vi "Plot Speed of Sound Freshwater.vi"() -> ()   [LabVIEW 2016]
uses:
  <vilib>/Analysis/1siggen.llb/Ramp Pattern by Samples.vi
  <vilib>/Analysis/NI_AALBase.lvlib
panel:
  in  "Stop Button":bool
  out "Speed of Sound":T1(graph)
  in  "Step[C]":dbl=0.1 min=0.0 max=100.0 step=0.1
  in  "High Temp [C]":dbl=70.0
  in  "Low Temp [C]":dbl
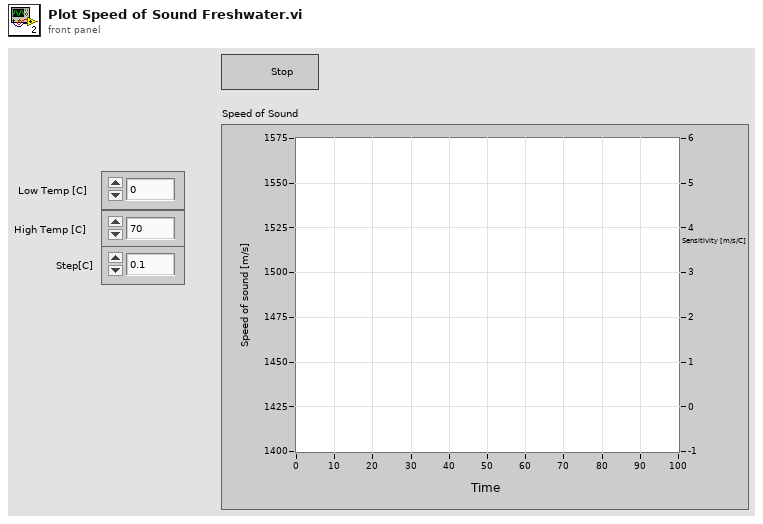
[diagram p1: front panel]
types:
  T1 = cluster{"Low Temp [C]":dbl, "Step[C]":dbl, "Sensitivity [m/s/C]":dbl[]}[]
  T2 = cluster{"Low Temp [C]":dbl, "Step[C]":dbl, "Speed of Sound [m/s]":dbl[]}
  T3 = cluster{"Low Temp [C]":dbl, "Step[C]":dbl, "Sensitivity [m/s/C]":dbl[]}
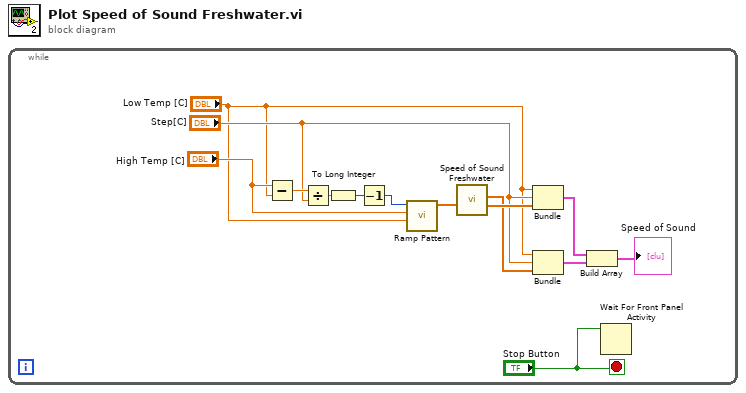
[diagram p0: block diagram]
diagram:
  n1 = while {
    stop <- "Stop Button" stop-if-true
    n2 = Subtract(x="High Temp [C]", y="Low Temp [C]") -> (x-y=w13:dbl)
    n3 = Divide(x=w13, y="Step[C]") -> (x/y=w11:dbl)
    n4 = To Long Integer(number=w11) -> (32bit integer=w10:i32)
    n5 = Decrement(x=w10) -> (x-1=w12:i32)
    n6 = call-poly <vilib>:"Ramp Pattern.vi"("start"="Low Temp [C]", "end"="High Temp [C]", "samples"=w12) -> ("Ramp Pattern"=w9:dbl[])  [unwired: 7 in, 1 out]
    n7 = call "Speed of Sound Freshwater.vi"("Temperatures [C]"=w9) -> ("Speed of Sound [m/s]"=w7:dbl[], "Sensitivity [m/s/C]"=w4:dbl[])  [unwired: 8 in, 1 out]
    n8 = Bundle("Low Temp [C]"="Low Temp [C]", "Step[C]"="Step[C]", "Speed of Sound [m/s]"=w7) -> (w3:T2)  [unwired: 1 in]
    n9 = Bundle("Low Temp [C]"="Low Temp [C]", "Step[C]"="Step[C]", "Sensitivity [m/s/C]"=w4) -> (w2:T3)  [unwired: 1 in]
    n10 = Build Array(w3, w2) -> (→"Speed of Sound":T1)
    n11 = Wait For Front Panel Activity(3:"Stop Button") -> ()  [unwired: 2 in, 1 out]
  }
